vi "Set Gas.vi"(8 "error in":errorcluster, 11 "Alicat in":refnum<class "Alicat.lvclass">) -> (0 "error out":errorcluster, 2 "String":string, 3 "Alicat out":refnum<class "Alicat.lvclass">)   [LabVIEW 2014, in "Alicat.lvlib" / "Alicat.lvclass"]
doc: "Return a string which may be readable by the Alicat device to set the operating gas."
uses:
  Alicat.lvclass
  Read Address.vi
  Read Gas.vi
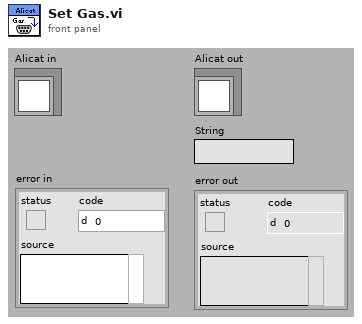
[diagram p1: front panel]
types:
  T1 = typedef "Untitled Library 2/Alicat.lvclass/Gas.ctl" = enum16{"Air", "Ar", "CH4", "CO", "CO2", "C2H6", "H2", "He", "N2", "NO", "Ne", "O2", "C3H8", "n-C4H10", "C2H2", "C2H4", "i-C2H10", "Kr", "Xe"}
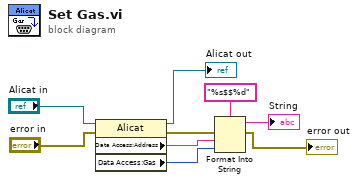
[diagram p0: block diagram]
diagram:
  n1 = property class="Alicat"(reference="Alicat in", error in="error in") -> (reference out=→"Alicat out":refnum<class "Alicat.lvclass">, error out=w2:errorcluster, "Data Access:Address"=w5:string, "Data Access:Gas"=w4:T1)
  n2 = Format Into String(format string="%s$$%d", error in=w2, w5, w4) -> (resulting string=→"String":string, error out=→"error out":errorcluster)  [unwired: 1 in]
